vi "get type info.vi"(11 "Type in":T1) -> (0 "Offset":u16, 1 "Group GUID":string, 2 "Type GUID":string, 3 "Starting Address Tag":string)   [LabVIEW 2015, in "Modbus Master System Explorer.lvlib"]
uses:
  Modbus Master System Explorer.lvlib
  Modbus Type.ctl
  Shared/Constants.vi
  Shared/Modbus Master Shared.lvlib
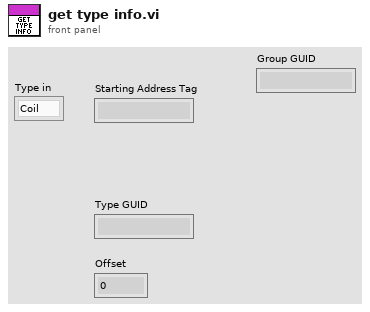
[diagram p1: front panel]
types:
  T1 = typedef "Modbus Master Shared.lvlib/Modbus Type.ctl" = enum16{"Coil", "Discrete Input", "Holding Register", "Input Register"}
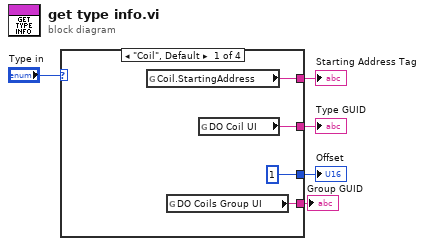
[diagram p0: block diagram]
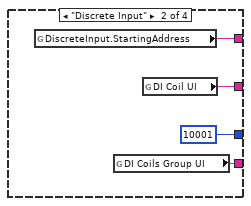
[diagram p2: hidden frame]
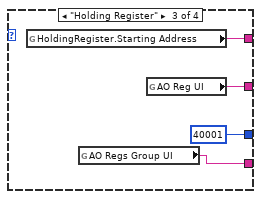
[diagram p3: hidden frame]
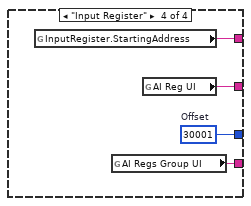
[diagram p4: hidden frame]
diagram:
  n1 = case shown="\"Coil\", Default" "Type in" {
    tunnel: [w9 w13 w17 w21] -> w3
    tunnel: [w8 w12 w16 w20] -> w2
    tunnel: [u16 1 ("Offset") u16 10001 ("Offset") u16 40001 ("Offset") w19] -> w5
    tunnel: [w6 w10 w14 w18] -> w1
    frame "Coil", Default {
      n2 = global read "Constants.vi" "Coil.StartingAddress"() -> (w8:string)
      n3 = global read "Constants.vi" "DO Coils Group UI"() -> (w6:string)
      n4 = global read "Constants.vi" "DO Coil UI"() -> (w9:string)
    }
    frame "Discrete Input" {
      n5 = global read "Constants.vi" "DiscreteInput.StartingAddress"() -> (w12:string)
      n6 = global read "Constants.vi" "DI Coils Group UI"() -> (w10:string)
      n7 = global read "Constants.vi" "DI Coil UI"() -> (w13:string)
    }
    frame "Holding Register" {
      n8 = global read "Constants.vi" "HoldingRegister.Starting Address"() -> (w16:string)
      n9 = global read "Constants.vi" "AO Regs Group UI"() -> (w14:string)
      n10 = global read "Constants.vi" "AO Reg UI"() -> (w17:string)
    }
    frame "Input Register" {
      w19 = u16 30001  # Offset
      n11 = global read "Constants.vi" "InputRegister.StartingAddress"() -> (w20:string)
      n12 = global read "Constants.vi" "AI Regs Group UI"() -> (w18:string)
      n13 = global read "Constants.vi" "AI Reg UI"() -> (w21:string)
    }
  }
  "Offset" <- w5
  "Type GUID" <- w3
  "Starting Address Tag" <- w2
  "Group GUID" <- w1
